vi "TLMotorStartCtrl.vi"(4 "Error In (No Error)":errorcluster, 6 "SerialNum":i32, 7 "Motor Ref":refnum<k7>) -> (0 "Error Out":errorcluster, 3 "Motor Ref":refnum<k7>)   [LabVIEW 2014]
doc: "Starts the Motor control.\n\nIn\nMotor Ref - Reference to Motor control object.\nError In (No Error) - Standard LabView error cluster.\n\nOut\nMotor Ref - Reference to Motor control object.\nError Out - Standard LabView error cluster."
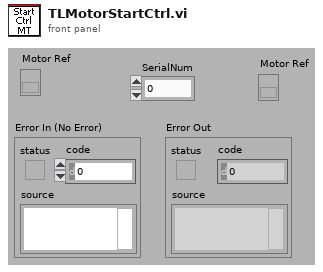
[diagram p1: front panel]
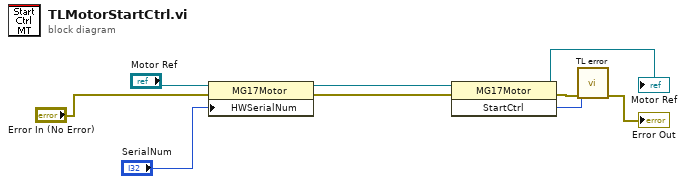
[diagram p0: block diagram]
diagram:
  n1 = property class="MG17Motor"(reference="Motor Ref", error in="Error In (No Error)", "HWSerialNum"="SerialNum") -> (reference out=w4:refnum<k7>, error out=w1:errorcluster)
  n2 = invoke class="MG17Motor" method="StartCtrl"(reference=w4, error in=w1) -> (reference out=→"Motor Ref":refnum<k7>, error out=w9:errorcluster, "StartCtrl"=w8:i32)  [unwired: 1 in]
  n3 = call "TL error.vi"("error in (no error)"=w9, "Return Code"=w8) -> ("error out"=→"Error Out":errorcluster)  [unwired: 9 in]
